vi "Apply Voltage.vi"(8 "error in (no error)":errorcluster, 11 "Tool Path in":refnum<class "Tool Path.lvclass">) -> (0 "error out":errorcluster, 3 "Tool Path out":refnum<class "Tool Path.lvclass">)   [LabVIEW 2019, in "Tool Path.lvclass"]
uses:
  Tool Path.lvclass
  Settings/ObjectSettings/ObjectSettings.lvclass/ObjectSettings.ctl
  Settings/Path Settings/Path Settings.lvclass
  C:/Users/Albro/Documents/GitHub/AFM-Lithography/lvsrc/Classes/Settings/ObjectSettings/ObjectSettings.lvclass
  Settings/ObjectSettings/ObjectSettings.lvclass
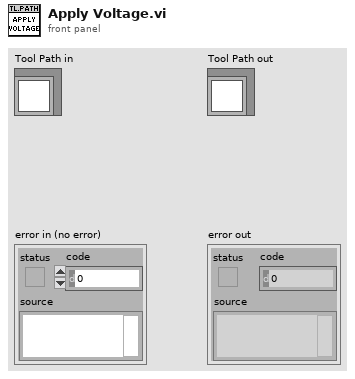
[diagram p1: front panel]
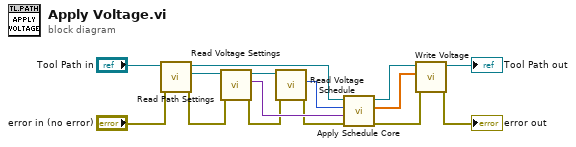
[diagram p0: block diagram]
diagram:
  n1 = call-dynamic "Read Path Settings.vi"("error in (no error)"="error in (no error)", "Tool Path in"="Tool Path in") -> ("error out"=w3:errorcluster, "Path Settings.lvclass"=w11:refnum<class "Path Settings.lvclass">, "Tool Path out"=w5:refnum<class "Tool Path.lvclass">)  [unwired: 7 in]
  n2 = call "Read Voltage Settings.vi"("error in (no error)"=w3, "ObjectSettings in"=w11) -> ("error out"=w2:errorcluster, "Settings"=w9:variant, "ObjectSettings out"=w10:refnum<class "Path Settings.lvclass">)  [unwired: 7 in]
  n3 = call "Read Voltage Schedule.vi"("error in (no error)"=w2, "ObjectSettings in"=w10) -> ("error out"=w7:errorcluster, "Schedule"=w8:u16)  [unwired: 7 in, 1 out]
  n4 = call-dynamic "Apply Schedule Core.vi"("error in (no error)"=w7, "Settings"=w9, "Schedule"=w8, "Tool Path in"=w5) -> ("error out"=w6:errorcluster, "Schedule Array"=w1:dbl[], "Tool Path out"=w4:refnum<class "Tool Path.lvclass">)  [unwired: 5 in]
  n5 = call-dynamic "Write Voltage.vi"("error in (no error)"=w6, "Voltage"=w1, "Tool Object in"=w4) -> ("error out"=→"error out":errorcluster, "Tool Object out"=→"Tool Path out":refnum<class "Tool Path.lvclass">)  [unwired: 7 in]
